vi "Actor Core.vi"(8 "error in":errorcluster, 11 "Nested in":refnum<class "USD Actor.lvclass">) -> (0 "error out":errorcluster, 3 "Actor out":refnum<class "Actor.lvclass">)   [LabVIEW 2019, in "USD Actor.lvlib" / "USD Actor.lvclass"]
doc: "(<B>Filename</B>: Actor Framework.lvlib:Actor.lvclass:Actor Core.vi)\n\nReceives messages to the actor, reacts to them, and initiates any error handling that may shut the actor down.\n\nDescendant classes may override this VI to append parallel tasks for the actor to complete while it handles messages. Overrides use the Call Parent Method node."
uses:
  USD Actor.lvclass
  C:/Program Files (x86)/National Instruments/LabVIEW 2019/vi.lib/ActorFramework/Actor/Actor.lvclass
  <vilib>/ActorFramework/Actor/Actor.lvclass
  <vilib>/ActorFramework/Actor/Actor.lvclass/Actor.ctl
  <vilib>/ActorFramework/Message Enqueuer/Message Enqueuer.lvclass/Message Enqueuer.ctl
  USD Actor.lvclass/USD Actor.ctl
  <vilib>/ActorFramework/Message Enqueuer/Init from Existing Queue.vi
  <vilib>/ActorFramework/Message Enqueuer/Enqueue.vi
  <vilib>/ActorFramework/Stop Msg/Stop Msg.lvclass
  C:/Program Files (x86)/National Instruments/LabVIEW 2019/vi.lib/ActorFramework/Message/Message.lvclass
  <vilib>/ActorFramework/Message Priority Queue/Priority Enqueue.vi
  <vilib>/ActorFramework/Message Enqueuer/Message Enqueuer.lvclass
  USD Actor Messages/Actualizar Credito Msg/Actualizar Credito Msg.lvclass
panel:
  in  "COIN 1":bool
  in  "COIN 2":bool
  in  "COIN 3":bool
  in  "COIN 4":bool
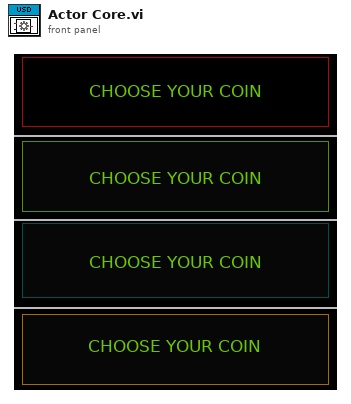
[diagram p1: front panel]
types:
  T1 = cluster{"[0]":bool, "[1]":bool, "[2]":bool, "[3]":bool}
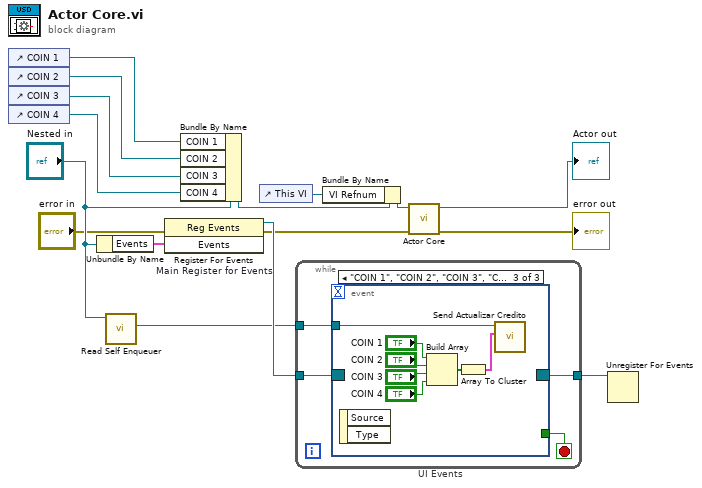
[diagram p0: block diagram]
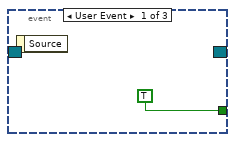
[diagram p2: hidden frame]
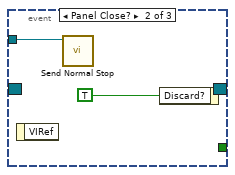
[diagram p3: hidden frame]
diagram:
  n1 = control-ref of="COIN 1"() -> (w4:refnum<vi>)
  n2 = control-ref of="COIN 2"() -> (w1:refnum<vi>)
  n3 = control-ref of="COIN 3"() -> (w2:refnum<vi>)
  n4 = control-ref of="COIN 4"() -> (w3:refnum<vi>)
  n5 = Unbundle By Name("Nested in") -> ("Events"=w13:cluster{"Stop":refnum<user-event>})
  n6 = call <vilib>:"Read Self Enqueuer.vi"("Actor"="Nested in") -> ("Self Enqueuer"=w10:refnum<class "Message Enqueuer.lvclass">)  [unwired: 10 in]
  n7 = register-events "Main Register for Events"(error in="error in", w13) -> (reference out=w14:refnum<event-registration>, error out=w8:errorcluster)  [unwired: 1 in]
  n8 = Bundle By Name(cluster="Nested in", "COIN 1"=w4, "COIN 2"=w1, "COIN 3"=w2, "COIN 4"=w3) -> (w5:refnum<class "USD Actor.lvclass">)
  n9 = control-ref of="This VI"() -> (w6:refnum<vi>)
  n10 = while {
    tunnel: w14 -> [w20]
    tunnel: [w18] -> w12
    tunnel: w10 -> [w17]
    stop <- w19 stop-if-true
    n11 = event "UI Events" shown="[2] \"COIN 1\", \"COIN 2\", \"COIN 3\", \"COIN 4\": Value Change" {
      selector: w20 -> [_ _ _]
      dyn-events: [_ _ _] -> w18
      timeout: _ -> [_ _ _]
      tunnel: [TRUE _ _] -> w19
      tunnel: w17 -> [_ w22 w25]
      event User Event {
        n12 = event-data() -> ()  [unwired: 1 in, 1 out]
      }
      event Panel Close? {
        n13 = event-data() -> ()  [unwired: 1 in, 1 out]
        n14 = call <vilib>:"Send Normal Stop.vi"("Message Enqueuer"=w22) -> ()  [unwired: 10 in, 1 out]
        n15 = event-data("Discard?"=TRUE) -> ()  [unwired: 1 in, 1 out]
      }
      event "COIN 1", "COIN 2", "COIN 3", "COIN 4": Value Change {
        n16 = event-data() -> ()  [unwired: 1 in, 2 out]
        n17 = Build Array("COIN 1", "COIN 2", "COIN 3", "COIN 4") -> (w26:bool[])
        n18 = Array To Cluster(array=w26) -> (cluster=w24:T1)
        n19 = call "Send Actualizar Credito.vi"("Cluster"=w24, "Message Enqueuer"=w25) -> ()  [unwired: 8 in, 2 out]
      }
    }
  }
  n20 = Bundle By Name(cluster=w5, "VI Refnum"=w6) -> (w7:refnum<class "USD Actor.lvclass">)
  n21 = call-parent "Actor Core.vi"("error in"=w8, "Actor in"=w7) -> ("error out"=→"error out":errorcluster, "Actor out"=→"Actor out":refnum<class "Actor.lvclass">)  [unwired: 8 in]
  n22 = Unregister For Events(event registration refnum=w12) -> ()  [unwired: 1 in, 1 out]
